vi "Setup MFC Outputs (SubVI).vi"(9 "task In":refnum<k21>, 10 "Array of Clusters Out":T1(array[cluster]), 11 "Array":tag[](array[tag])) -> (0 "error out":errorcluster, 3 "Refnum out":refnum<k21>)   [LabVIEW 2011]
uses:
  <vilib>/Utility/error.llb/DialogType.ctl
  <vilib>/DAQmx/create/channels.llb/DAQmx Create Channel (AO-Voltage-Basic).vi
  Program Files (x86)/National Instruments/LabVIEW 2011/resource/objmgr/daqmx.rc
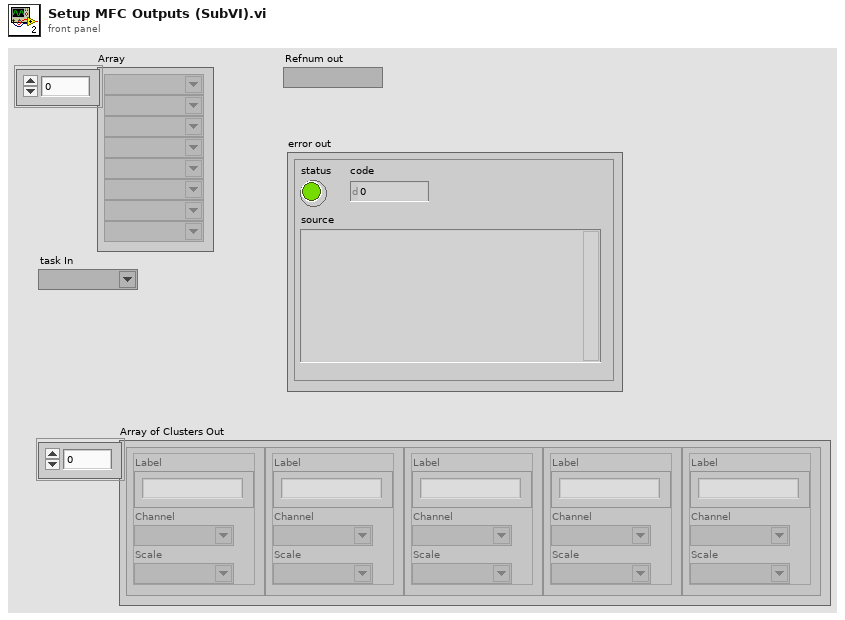
[diagram p1: front panel]
types:
  T1 = cluster{"Label":string, "Channel":tag, "Scale":tag}[]
  T2 = typedef "DialogType.ctl" = u16
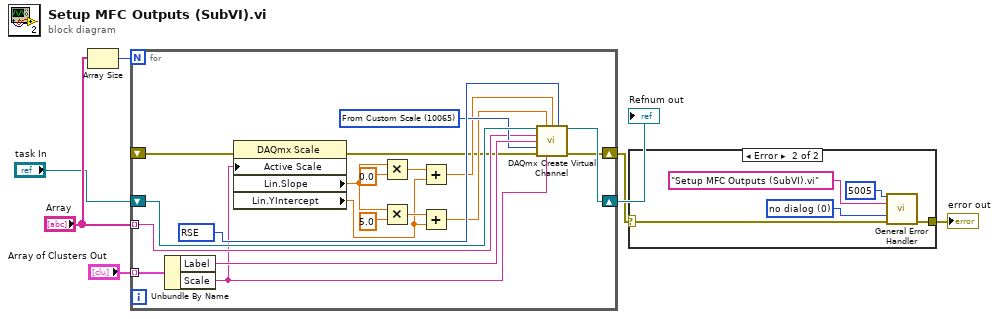
[diagram p0: block diagram]
diagram:
  n1 = Array Size(array="Array") -> (size(s)=w4:i32)
  n2 = for {
    N: w4 -> [_]
    tunnel: "Array" -> [w20] mode=indexing
    shift-right: [w26] -> w7
    shift-left: "task In" -> [w25]
    shift-right: [w8] -> w1
    shift-left: _ -> [w18]
    tunnel: "Array of Clusters Out" -> [w23] mode=indexing
    w21 = 10065 items=["Volts"=10348, "From Custom Scale"=10065] ("units")
    w24 = 10083 items=["Default"=-1, "RSE"=10083, "Differential"=10106, "Pseudodifferential"=12529] ("output terminal configuration")
    n3 = Unbundle By Name(w23) -> ("Label"=w22:string, "Scale"=w19:tag)
    n4 = property class="DAQmx Scale"(error in=w18, "Active Scale"=w19) -> (error out=w9:errorcluster, "Lin.Slope"=w13:dbl, "Lin.YIntercept"=w12:dbl)  [unwired: 1 in, 1 out]
    n5 = Multiply(x=w13, y=0.0) -> (x*y=w16:dbl)
    n6 = Multiply(x=w13, y=5.0) -> (x*y=w15:dbl)
    n7 = Add(x=w16, y=w12) -> (x+y=w11:dbl)
    n8 = Add(x=w15, y=w12) -> (x+y=w10:dbl)
    n9 = call-poly <vilib>:"DAQmx Create Virtual Channel.vi"("task in"=w25, "maximum value"=w10, "minimum value"=w11, "output terminal configuration"=w24, "physical channels"=w20, "name to assign"=w22, "units"=w21, "error in"=w9, "custom scale name"=w19) -> ("task out"=w26:refnum<k21>, "error out"=w8:errorcluster)  [unwired: 5 in]
  }
  "Refnum out" <- w7
  n10 = case shown="Error" w1 {
    selector: w1 -> [w27 w32]
    tunnel: [w27 w31] -> w2
    frame No Error {
    }
    frame Error {
      w28 = T2 0 items=["no dialog", "OK message", "continue or stop message", "OK message + warnings", "continue/stop + warnings"] ("type of dialog (OK msg:1)")
      n11 = call <vilib>:"General Error Handler.vi"("[error code] (0)"=5005, "[error source] (\" \")"="Setup MFC Outputs (SubVI).vi" ("[error source] (\" \")"), "type of dialog (OK msg:1)"=w28, "error in (no error)"=w32) -> ("error out"=w31:errorcluster)  [unwired: 7 in, 4 out]
    }
  }
  "error out" <- w2
